vi "generator_init.vi"(8 "error in (no error)":errorcluster, 11 "VISA Refnum in":refnum<visa-resource-name>) -> (0 "error out":errorcluster, 3 "VISA Refnum out":refnum<visa-resource-name>)   [LabVIEW 2022 SP3]
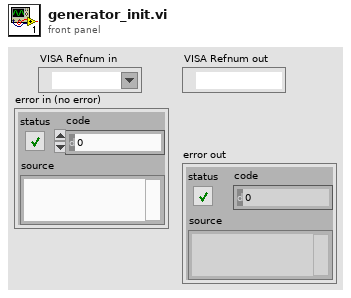
[diagram p1: front panel]
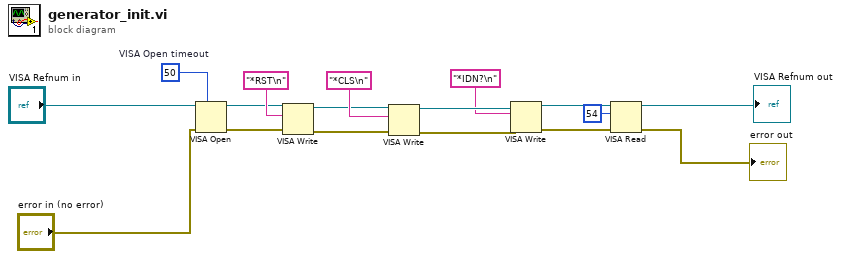
[diagram p0: block diagram]
diagram:
  w7 = u32 50  # VISA Open timeout
  n1 = VISA Open(timeout (0)=w7, error in (no error)="error in (no error)", VISA resource name="VISA Refnum in") -> (VISA resource name=w11:refnum<visa-resource-name>, error out=w10:errorcluster)  [unwired: 2 in]
  n2 = VISA Write(VISA resource name=w11, write buffer="*RST\n", error in (no error)=w10) -> (VISA resource name out=w13:refnum<visa-resource-name>, error out=w14:errorcluster)  [unwired: 1 out]
  n3 = VISA Write(VISA resource name=w13, write buffer="*CLS\n", error in (no error)=w14) -> (VISA resource name out=w16:refnum<visa-resource-name>, error out=w17:errorcluster)  [unwired: 1 out]
  n4 = VISA Write(VISA resource name=w16, write buffer="*IDN?\n", error in (no error)=w17) -> (VISA resource name out=w4:refnum<visa-resource-name>, error out=w5:errorcluster)  [unwired: 1 out]
  n5 = VISA Read(VISA resource name=w4, byte count=u32 54, error in (no error)=w5) -> (VISA resource name out=→"VISA Refnum out":refnum<visa-resource-name>, error out=→"error out":errorcluster)  [unwired: 2 out]
